vi "PH_SRDG645.panel.vi"(0 "object ref":refnum<vi>, 5 "error in (no error)":errorcluster) -> (19 "error out":errorcluster)   [LabVIEW 2014, in "PH_SRDG645.lvlib"]
doc: "By this VI an ignitron can be monitored and switched. \n\n\"HEATING ON\" and \"WATER ON\" indicate the status (blue: bad tag value, no connection, or internal problems; lightgreen: on; red: off).\n\nThe button switches the electronic of the ignitron, \"SWITCH STATE\" indicates the switch status (blue: bad tag value, no connection, or internal problems; darkgreen: off; lightgreen: on).\n\n\"TRIGGER\" and \"TRIGGER PULSE\" indicate the status of the trigger (blue: bad tag value, no connection, or internal problems; darkgreen: off; lightgreen: on).\n\n\"on since\" indicates at which time the Ignition has been switched on.\n\n\"EXIT\" closes the front panel (GUI), while \"Delete Instance\" disconnects and removes the instance from the PCS.\n\nThis VI has no machine safety relevant logig: there is neither a check of internal conclict nor with other objects. Therefore it must be handled with care and should be operated by well educated operators only. It is forseen exclusively for direct operating and testing of the system. \n\nLicense Agreement for this software:\n\nCopyright (C)\nGesellschaft für Schwerionenforschung, GSI\nPlanckstr. 1\n64291 Darmstadt\nGermany\n\nContact: D.Beck@gsi.de \n\nThis program is free software; you can redistribute it and/or modify it under the terms of the GNU General Public License as published by the Free Software Foundation; either version 2 of the license, or (at your option) any later version.\n\nThis program is distributed in the hope that it will be useful, but WITHOUT ANYW ARRANTY; without even the implied warranty of MERCHANTABILITY or FITNESS FOR A PARTICULAR PURPOSE. See the GNU General License for more details (http://www.gnu.org).\n\nGesellschaft für Schwerionenforschung, GSI\nPlanckstr. 1, 64291 Darmstadt, Germany\nFor all questions and ideas contact: M.Richter@gsi.de, H.Brand@gsi.de or D.Beck@gsi.de.\nLast update: 18-DEC-2002"
uses:
  PH_SRDG645.lvlib
  PH_StatusHandler/PH_StatusHandler.GUI element.ctl
  PH_SRDG645.Trigger.ctl
  PH_SRDG645.Channel Settings.ctl
  PH_SRDG645.Output Settings.ctl
  instr.lib/Stanford Research DG645/Driver/Output BNC.ctl
  instr.lib/Stanford Research DG645/Driver/Channel.ctl
  CSCore/CSObj/CSObj.lvlib
  PH_Common/PH_Common.lvlib
  CSCore/CSSystem/CSSystemLib/CSSystemLib.lvlib
  instr.lib/Stanford Research DG645/Stanford Research DG645 - Driver.lvlib
  PH_Class/PH_Class.lvlib
  PH_PSDBWriter/PH_PSDBWriter.lvlib
  PH_StatusHandler/PH_StatusHandler.lvlib
panel:
  out "PSDB Status":u32(colorbox)=6618880 caption="PSDB"
  in  "Tab Control":T1(tab)
  in  "H":T2 {"relative to" items=["T0", "T1", "A", "B", "C", "D", "E", "F", "G", "H"]; "Delay [s]" format="%#_12p"}
  in  "G":T2 {"relative to" items=["T0", "T1", "A", "B", "C", "D", "E", "F", "G", "H"]; "Delay [s]" format="%#_12p"}
  in  "F":T2 {"relative to" items=["T0", "T1", "A", "B", "C", "D", "E", "F", "G", "H"]; "Delay [s]" format="%#_12p"}
  in  "E":T2 {"relative to" items=["T0", "T1", "A", "B", "C", "D", "E", "F", "G", "H"]; "Delay [s]" format="%#_12p"}
  in  "D":T2 {"relative to" items=["T0", "T1", "A", "B", "C", "D", "E", "F", "G", "H"]; "Delay [s]" format="%#_12p"}
  in  "C":T2 {"relative to" items=["T0", "T1", "A", "B", "C", "D", "E", "F", "G", "H"]; "Delay [s]" format="%#_12p"}
  in  "B":T2 {"relative to" items=["T0", "T1", "A", "B", "C", "D", "E", "F", "G", "H"]; "Delay [s]" format="%#_12p"}
  in  "A":T2 {"relative to" items=["T0", "T1", "A", "B", "C", "D", "E", "F", "G", "H"]; "Delay [s]" format="%#_12p"}
  in  "T1":T2 {"relative to" items=["T0", "T1", "A", "B", "C", "D", "E", "F", "G", "H"]; "Delay [s]" format="%#_12p"}
  in  "T0":T3 {"Polarity" items=["negative", "positive"]}
  in  "GH":T3 {"Polarity" items=["negative", "positive"]}
  in  "EF":T3 {"Polarity" items=["negative", "positive"]}
  in  "CD":T3 {"Polarity" items=["negative", "positive"]}
  in  "AB":T3 {"Polarity" items=["negative", "positive"]}
  in  "Trigger Settings":T4={"Source"=0, "Rate [Hz]"=1000.0, "Level [V]"=1.0} {"Rate [Hz]" format="%#_9p"; "Source" items=["Internal", "External rising edge", "External falling edge", "Single shot external rising edges", "Single shot external falling edges", "Single shot", "Line"]}
  in  "Get Hardware Settings":bool
  out "Model":string
  out "Serial Number":string
  out "Firmware Revision":string
  out "Default Name":string
  out "Device Errors":cluster{"code":i32, "Text":string}[](array[cluster])
  out "VISA Resource":string
  out "Status":T5 caption="Enabling State"
  in  "Delete":bool
  in  "Exit":bool
  out "loop counter":i32
  # "PCS"
  # "3.40"
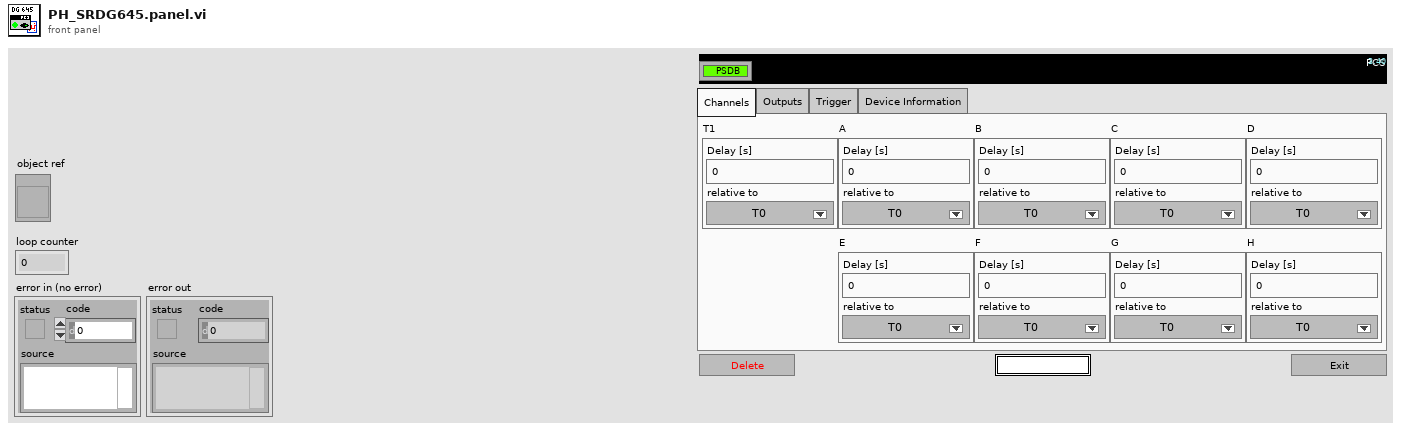
[diagram p1: front panel]
types:
  T1 = enum32{"Channels", "Outputs", "Trigger", "Device Information"}
  T2 = typedef "PH_SRDG645.lvlib/PH_SRDG645.Channel Settings.ctl" = cluster{"Delay [s]":dbl, "relative to":i32}
  T3 = typedef "PH_SRDG645.lvlib/PH_SRDG645.Output Settings.ctl" = cluster{"Level Offset [V]":dbl, "Amplitue [V]":dbl, "Polarity":i32}
  T4 = typedef "PH_SRDG645.lvlib/PH_SRDG645.Trigger.ctl" = cluster{"Source":i32, "Rate [Hz]":dbl, "Level [V]":dbl}
  T5 = typedef "PH_StatusHandler.lvlib/PH_StatusHandler.GUI element.ctl" = u16
  T6 = typedef "Stanford Research DG645 - Driver.lvlib/Output BNC.ctl" = i32
  T7 = typedef "Stanford Research DG645 - Driver.lvlib/Channel.ctl" = i32
  T8 = typedef "PH_SRDG645.lvlib/PH_SRDG645.i attribute.ctl" = cluster{"GUI Refs":cluster{"Delete":refnum<vi>, "Device Errors":refnum<vi>, "Trigger":refnum<vi>, "Default Name":refnum<vi>, "Firmware Revision":refnum<vi>, "Serial Number":refnum<vi>, "Model":refnum<vi>, "Visa resource name":refnum<vi>}, "Service ID Rate":i32, "Service IDs Channelinfo":i32[], "VISA resource name":refnum<visa-resource-name>, "Device Errors":cluster{"code":i32, "Text":string}[], "Trigger":T4, "Channels":cluster{"T1":T2, "A":T2, "B":T2, "C":T2, "D":T2, "E":T2, "F":T2, "G":T2, "H":T2}, "GUI Refs Channels":refnum<vi>[], "Outputs":cluster{"AB":cluster{"Level Offset [V]":dbl, "Amplitue [V]":dbl, "Polarity":i32}, "CD":cluster{"Level Offset [V]":dbl, "Amplitue [V]":dbl, "Polarity":i32}, "EF":cluster{"Level Offset [V]":dbl, "Amplitue [V]":dbl, "Polarity":i32}, "GH":cluster{"Level Offset [V]":dbl, "Amplitue [V]":dbl, "Polarity":i32}, "T0":cluster{"Level Offset [V]":dbl, "Amplitue [V]":dbl, "Polarity":i32}}, "GUI Refs Outputs":refnum<vi>[], "Serial Number":string, "Firmweare Revision":string, "Model":string}
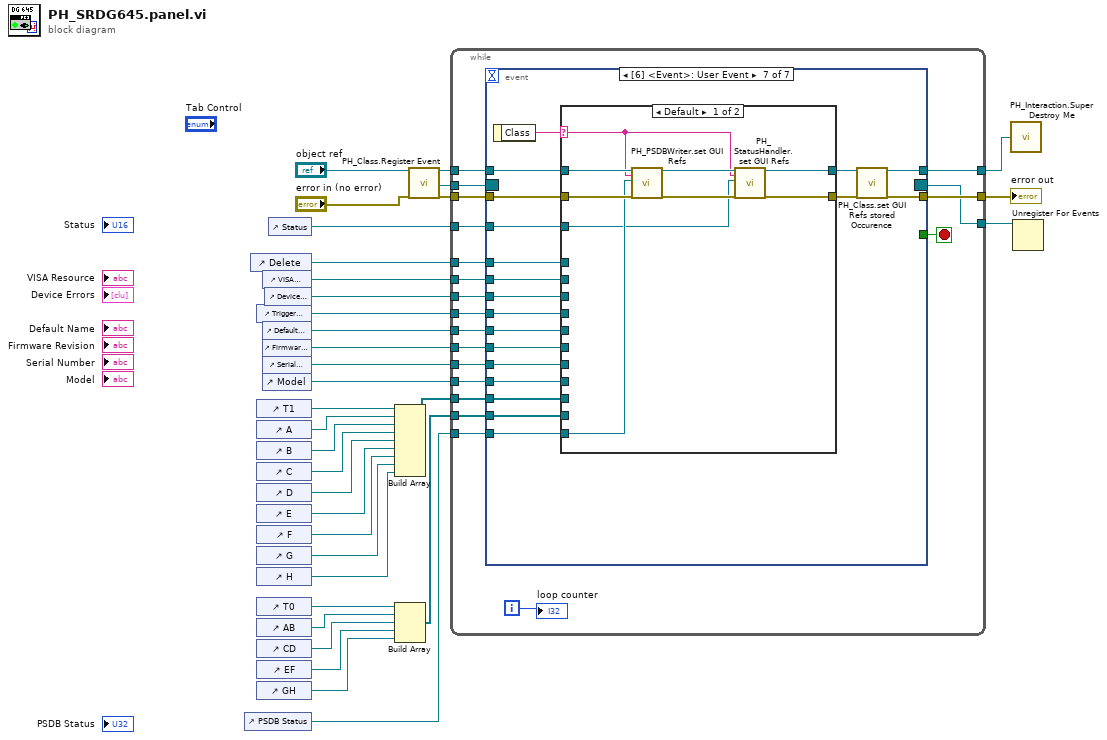
[diagram p0: block diagram]
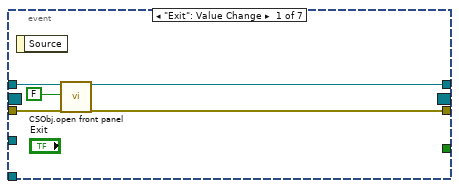
[diagram p2: hidden frame]
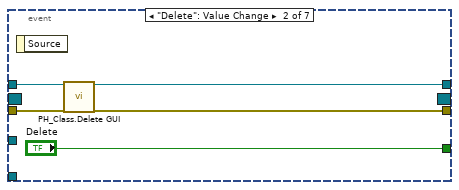
[diagram p3: hidden frame]
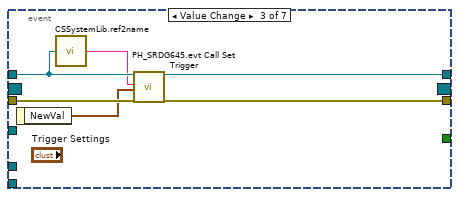
[diagram p4: hidden frame]
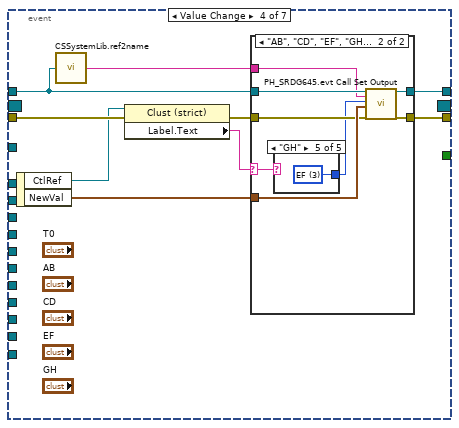
[diagram p5: hidden frame]
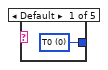
[diagram p7: hidden frame]
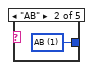
[diagram p8: hidden frame]
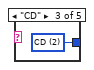
[diagram p9: hidden frame]
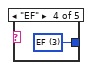
[diagram p10: hidden frame]
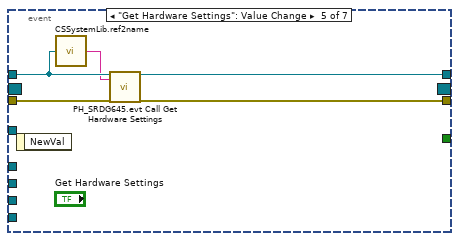
[diagram p11: hidden frame]
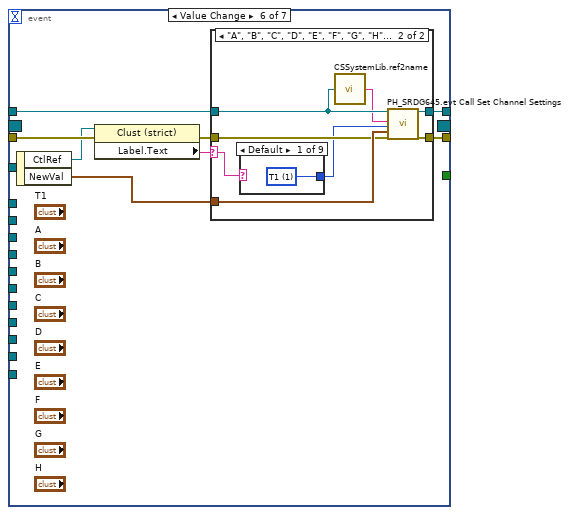
[diagram p12: hidden frame]
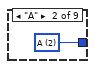
[diagram p14: hidden frame]
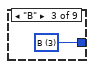
[diagram p15: hidden frame]
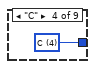
[diagram p16: hidden frame]
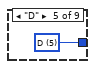
[diagram p17: hidden frame]
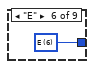
[diagram p18: hidden frame]
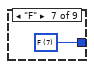
[diagram p19: hidden frame]
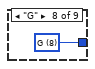
[diagram p20: hidden frame]
diagram:
  n1 = control-ref of="PSDB Status"() -> (w14:refnum<vi>)
  n2 = control-ref of="Delete"() -> (w11:refnum<vi>)
  n3 = control-ref of="Trigger Settings"() -> (w8:refnum<vi>)
  n4 = control-ref of="T1"() -> (w32:refnum<vi>)
  n5 = control-ref of="A"() -> (w31:refnum<vi>)
  n6 = control-ref of="B"() -> (w30:refnum<vi>)
  n7 = control-ref of="C"() -> (w29:refnum<vi>)
  n8 = control-ref of="D"() -> (w28:refnum<vi>)
  n9 = control-ref of="E"() -> (w27:refnum<vi>)
  n10 = control-ref of="F"() -> (w26:refnum<vi>)
  n11 = control-ref of="G"() -> (w25:refnum<vi>)
  n12 = control-ref of="H"() -> (w24:refnum<vi>)
  n13 = control-ref of="T0"() -> (w23:refnum<vi>)
  n14 = control-ref of="AB"() -> (w22:refnum<vi>)
  n15 = control-ref of="CD"() -> (w21:refnum<vi>)
  n16 = control-ref of="EF"() -> (w20:refnum<vi>)
  n17 = control-ref of="GH"() -> (w19:refnum<vi>)
  n18 = control-ref of="VISA Resource"() -> (w10:refnum<vi>)
  n19 = control-ref of="Default Name"() -> (w7:refnum<vi>)
  n20 = control-ref of="Firmware Revision"() -> (w6:refnum<vi>)
  n21 = control-ref of="Serial Number"() -> (w5:refnum<vi>)
  n22 = control-ref of="Model"() -> (w4:refnum<vi>)
  n23 = control-ref of="Device Errors"() -> (w9:refnum<vi>)
  n24 = control-ref of="Status"() -> (w1:refnum<vi>)
  n25 = Build Array(w32, w31, w30, w29, w28, w27, w26, w25, w24) -> (w3:refnum<vi>[])
  n26 = Build Array(w23, w22, w21, w20, w19) -> (w2:refnum<vi>[])
  n27 = call "PH_Class.Register Event.vi"("i ref in"="object ref", "error in (no error)"="error in (no error)") -> ("i ref out"=w18:refnum<vi>, "Event Registration Refnum"=w16:refnum<event-registration>, "error out"=w17:errorcluster)  [unwired: 15 in]
  n28 = while {
    tunnel: w18 -> [w50]
    tunnel: [w49] -> w34
    tunnel: w17 -> [w52]
    tunnel: [w51] -> w33
    tunnel: w16 -> [w48]
    tunnel: [w47] -> w15
    tunnel: w14 -> [w46]
    tunnel: w11 -> [w45]
    tunnel: w1 -> [w44]
    tunnel: w10 -> [w43]
    tunnel: w9 -> [w42]
    tunnel: w8 -> [w41]
    tunnel: w7 -> [w40]
    tunnel: w6 -> [w39]
    tunnel: w5 -> [w38]
    tunnel: w4 -> [w37]
    tunnel: w3 -> [w36]
    tunnel: w2 -> [w35]
    i -> [w53]
    stop <- w54 stop-if-true
    n29 = event shown="[6] <Event>: User Event" {
      selector: w48 -> [_ _ _ _ _ _ _]
      dyn-events: [_ _ _ _ _ _ _] -> w47
      timeout: _ -> [_ _ _ _ _ _ _]
      tunnel: [_ "Delete" _ _ _ _ _] -> w54
      tunnel: w50 -> [w59 w63 w66 w75 w97 w104 w143]
      tunnel: w52 -> [w57 w62 w69 w78 w95 w106 w141]
      tunnel: [w56 w61 w68 w77 w98 w105 w144] -> w51
      tunnel: [w55 w60 w70 w79 w99 w107 w145] -> w49
      tunnel: w46 -> [_ _ _ _ _ _ w138]
      tunnel: w45 -> [_ _ _ _ _ _ w137]
      tunnel: w44 -> [_ _ _ _ _ _ w136]
      tunnel: w43 -> [_ _ _ _ _ _ w135]
      tunnel: w42 -> [_ _ _ _ _ _ w134]
      tunnel: w41 -> [_ _ _ _ _ _ w133]
      tunnel: w40 -> [_ _ _ _ _ _ w132]
      tunnel: w39 -> [_ _ _ _ _ _ w131]
      tunnel: w38 -> [_ _ _ _ _ _ w130]
      tunnel: w37 -> [_ _ _ _ _ _ w129]
      tunnel: w36 -> [_ _ _ _ _ _ w128]
      tunnel: w35 -> [_ _ _ _ _ _ w127]
      event "Exit": Value Change {
        n30 = event-data() -> ()  [unwired: 1 in, 1 out]
        n31 = call "CSObj.open front panel.vi"("i ref in"=w59, "frontPanelOpen"=FALSE ("front panel open"), "error in (no error)"=w57) -> ("i ref out"=w55:refnum<vi>, "error out"=w56:errorcluster)  [unwired: 15 in]
      }
      event "Delete": Value Change {
        n32 = event-data() -> ()  [unwired: 1 in, 1 out]
        n33 = call "PH_Class.Delete GUI.vi"("VI in"=w63, "error in (no error)"=w62) -> ("VI out"=w60:refnum<vi>, "error out"=w61:errorcluster)  [unwired: 16 in]
      }
      event Value Change {
        n34 = event-data() -> ("NewVal"=w67:T4)  [unwired: 1 in]
        n35 = call "CSSystemLib.ref2name.vi"("obj refnum"=w66) -> ("name"=w65:string)
        n36 = call "PH_SRDG645.evt Call Set Trigger.vi"("i ref in"=w66, "Generator Instance"=w65, "Trigger Settings"=w67, "error IO"=w69) -> ("i ref out"=w70:refnum<vi>, "error out"=w68:errorcluster)  [unwired: 14 in]
      }
      event Value Change {
        n37 = event-data() -> ("CtlRef"=w72:refnum<vi>, "NewVal"=w76:T3)  [unwired: 1 in]
        n38 = call "CSSystemLib.ref2name.vi"("obj refnum"=w75) -> ("name"=w74:string)
        n39 = property class="Clust (strict)"(reference=w72, error in=w78) -> (error out=w73:errorcluster, "Label.Text"=w71:string)  [unwired: 1 out]
        n40 = case shown="\"AB\", \"CD\", \"EF\", \"GH\", \"T0\"" w71 {
          selector: w71 -> [_ w83]
          tunnel: [w81 w89] -> w79
          tunnel: [w80 w88] -> w77
          tunnel: w76 -> [_ w87]
          tunnel: w75 -> [w81 w86]
          tunnel: w74 -> [_ w85]
          tunnel: w73 -> [w80 w84]
          frame Default {
          }
          frame "AB", "CD", "EF", "GH", "T0" {
            n41 = case shown="\"GH\"" w83 {
              tunnel: [w90 w91 w92 w93 w94] -> w82
              frame Default {
                w90 = T6 0 items=["T0", "AB", "CD", "EF", "GH"] ("Output BNC")
              }
              frame "AB" {
                w91 = T6 1 items=["T0", "AB", "CD", "EF", "GH"] ("Output BNC")
              }
              frame "CD" {
                w92 = T6 2 items=["T0", "AB", "CD", "EF", "GH"] ("Output BNC")
              }
              frame "EF" {
                w93 = T6 3 items=["T0", "AB", "CD", "EF", "GH"] ("Output BNC")
              }
              frame "GH" {
                w94 = T6 3 items=["T0", "AB", "CD", "EF", "GH"] ("Output BNC")
              }
            }
            n42 = call "PH_SRDG645.evt Call Set Output.vi"("i ref in"=w86, "Generator Instance"=w85, "Output BNC"=w82, "Output Settings"=w87, "error IO"=w84) -> ("i ref out"=w89:refnum<vi>, "error out"=w88:errorcluster)  [unwired: 13 in]
          }
        }
      }
      event "Get Hardware Settings": Value Change {
        n43 = event-data() -> ()  [unwired: 1 in, 1 out]
        n44 = call "CSSystemLib.ref2name.vi"("obj refnum"=w97) -> ("name"=w96:string)
        n45 = call "PH_SRDG645.evt Call Get Hardware Settings.vi"("i ref in"=w97, "Generator Instance"=w96, "error IO"=w95) -> ("i ref out"=w99:refnum<vi>, "error out"=w98:errorcluster)  [unwired: 15 in]
      }
      event Value Change {
        n46 = event-data() -> ("CtlRef"=w101:refnum<vi>, "NewVal"=w103:T2)  [unwired: 1 in]
        n47 = property class="Clust (strict)"(reference=w101, error in=w106) -> (error out=w102:errorcluster, "Label.Text"=w100:string)  [unwired: 1 out]
        n48 = case shown="\"A\", \"B\", \"C\", \"D\", \"E\", \"F\", \"G\", \"H\", \"T1\"" w100 {
          selector: w100 -> [_ w110]
          tunnel: [w109 w117] -> w107
          tunnel: [w108 w116] -> w105
          tunnel: w104 -> [w109 w115]
          tunnel: w103 -> [_ w113]
          tunnel: w102 -> [w108 w112]
          frame Default {
          }
          frame "A", "B", "C", "D", "E", "F", "G", "H", "T1" {
            n49 = case shown="Default" w110 {
              tunnel: [w118 w119 w120 w121 w122 w123 w124 w125 w126] -> w111
              frame Default {
                w118 = T7 1 items=["T0", "T1", "A", "B", "C", "D", "E", "F", "G", "H"] ("Channel to set")
              }
              frame "A" {
                w119 = T7 2 items=["T0", "T1", "A", "B", "C", "D", "E", "F", "G", "H"] ("Channel to set")
              }
              frame "B" {
                w120 = T7 3 items=["T0", "T1", "A", "B", "C", "D", "E", "F", "G", "H"] ("Channel to set")
              }
              frame "C" {
                w121 = T7 4 items=["T0", "T1", "A", "B", "C", "D", "E", "F", "G", "H"] ("Channel to set")
              }
              frame "D" {
                w122 = T7 5 items=["T0", "T1", "A", "B", "C", "D", "E", "F", "G", "H"] ("Channel to set")
              }
              frame "E" {
                w123 = T7 6 items=["T0", "T1", "A", "B", "C", "D", "E", "F", "G", "H"] ("Channel to set")
              }
              frame "F" {
                w124 = T7 7 items=["T0", "T1", "A", "B", "C", "D", "E", "F", "G", "H"] ("Channel to set")
              }
              frame "G" {
                w125 = T7 8 items=["T0", "T1", "A", "B", "C", "D", "E", "F", "G", "H"] ("Channel to set")
              }
              frame "H" {
                w126 = T7 9 items=["T0", "T1", "A", "B", "C", "D", "E", "F", "G", "H"] ("Channel to set")
              }
            }
            n50 = call "CSSystemLib.ref2name.vi"("obj refnum"=w115) -> ("name"=w114:string)
            n51 = call "PH_SRDG645.evt Call Set Channel Settings.vi"("i ref in"=w115, "Generator Instance"=w114, "Channel to set"=w111, "Channel Settings"=w113, "error IO"=w112) -> ("i ref out"=w117:refnum<vi>, "error out"=w116:errorcluster)  [unwired: 13 in]
          }
        }
      }
      event User Event {
        n52 = event-data() -> ("Class"=w139:string)  [unwired: 1 in]
        n53 = case shown="Default" w139 {
          selector: w139 -> [w147 _]
          tunnel: w143 -> [w154 w168]
          tunnel: [w148 w167] -> w142
          tunnel: w141 -> [w153 w166]
          tunnel: [w150 w165] -> w140
          tunnel: w138 -> [w151 _]
          tunnel: w137 -> [_ w164]
          tunnel: w136 -> [w146 _]
          tunnel: w135 -> [_ w163]
          tunnel: w134 -> [_ w162]
          tunnel: w133 -> [_ w161]
          tunnel: w132 -> [_ w160]
          tunnel: w131 -> [_ w159]
          tunnel: w130 -> [_ w158]
          tunnel: w129 -> [_ w157]
          tunnel: w128 -> [_ w156]
          tunnel: w127 -> [_ w155]
          frame Default {
            n54 = call "PH_PSDBWriter.set GUI Refs.vi"("i ref in"=w154, "Class"=w147, "Ref PSDB Status"=w151, "error in"=w153) -> ("i ref out"=w149:refnum<vi>, "error out"=w152:errorcluster)  [unwired: 14 in]
            n55 = call "PH_StatusHandler.set GUI Refs.vi"("i ref in"=w149, "Class"=w147, "GUI Ref"=w146, "error in (no error)"=w152) -> ("i ref out"=w148:refnum<vi>, "error out"=w150:errorcluster)  [unwired: 14 in]
          }
          frame "PH_SRDG645" {
            n56 = call "PH_SRDG645.get data to modify.vi"("i ref in"=w168, "ms timeout (10000)"=-1, "error in (no error)"=w166) -> ("i ref out"=w173:refnum<vi>, "i attribute"=w171:T8, "error out"=w172:errorcluster)  [unwired: 13 in, 1 out]
            n57 = Bundle By Name(cluster=w171, "GUI Refs.Delete"=w164, "GUI Refs.Visa resource name"=w163, "GUI Refs.Device Errors"=w162, "GUI Refs.Trigger"=w161, "GUI Refs.Default Name"=w160, "GUI Refs.Firmware Revision"=w159, "GUI Refs.Serial Number"=w158, "GUI Refs.Model"=w157, "GUI Refs Channels"=w156, "GUI Refs Outputs"=w155) -> (w170:T8)
            n58 = call "PH_SRDG645.set modified data.vi"("i ref in"=w173, "i attribute"=w170, "error in (no error)"=w172) -> ("i ref out"=w167:refnum<vi>, "error out"=w165:errorcluster)  [unwired: 15 in]
          }
        }
        n59 = call "PH_Class.set GUI Refs stored Occurence.vi"("i ref in"=w142, "error in (no error)"=w140) -> ("i ref out"=w145:refnum<vi>, "error out"=w144:errorcluster)  [unwired: 16 in]
      }
    }
    "loop counter" <- w53
  }
  "error out" <- w33
  n60 = call "PH_Interaction.Super Destroy Me.vi"("i ref out"=w34) -> ()
  n61 = Unregister For Events(event registration refnum=w15) -> ()  [unwired: 1 in, 1 out]
